vi "Configure Calculation.vi"(4 "Upper Limit Value (0)":dbl format="%#_11g", 6 "Lower Limit Value (0)":dbl format="%#_11g", 7 "Enable Statistics (Disable)":bool, 8 "error in (no error)":errorcluster, 9 "Enable Limit Filter (Disable)":bool, 10 "N (100)":i32=100 min=2 max=1000000, 11 "VISA resource name":refnum<visa-resource-name>) -> (0 "error out":errorcluster, 3 "VISA resource name out":refnum<visa-resource-name>)   [LabVIEW 2020, in "Counter.lvlib" / "PICOTEST U62XXA series.lvlib"]
doc: "Configures settings required for post-acquisition Statistics computation.\n\n<B>Note:</B>\n\nTotalize and Volt Peak Measurements <B>does not</B> support post acquisiton Statistics computation."
uses:
  PICOTEST U62XXA series.lvlib
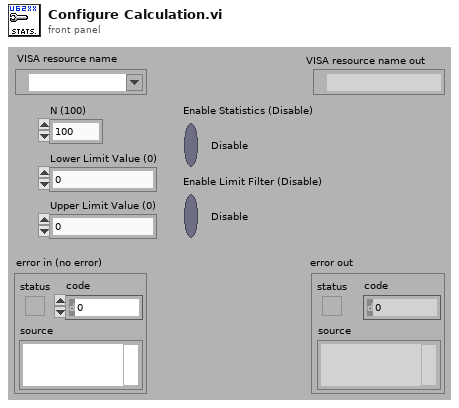
[diagram p1: front panel]
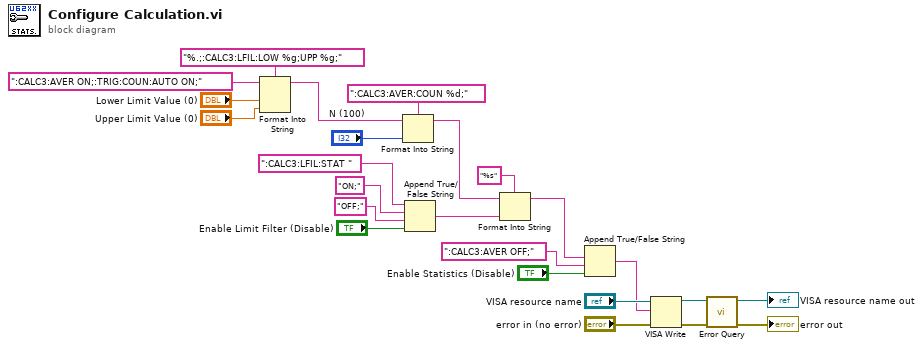
[diagram p0: block diagram]
diagram:
  n1 = Format Into String(format string="%.;:CALC3:LFIL:LOW %g;UPP %g;", initial string=":CALC3:AVER ON;:TRIG:COUN:AUTO ON;" ("format string"), "Lower Limit Value (0)", "Upper Limit Value (0)") -> (resulting string=w5:string)  [unwired: 1 in, 1 out]
  n2 = Format Into String(format string=":CALC3:AVER:COUN %d;", initial string=w5, "N (100)") -> (resulting string=w4:string)  [unwired: 1 in, 1 out]
  n3 = Append True/False String(1:"Enable Limit Filter (Disable)", 2:"OFF;" ("multi-line string"), 3:"ON;" ("multi-line string"), 4:":CALC3:LFIL:STAT " ("format string")) -> (0:w3:string)
  n4 = Format Into String(format string="%s", initial string=w4, w3) -> (resulting string=w1:string)  [unwired: 1 in, 1 out]
  n5 = Append True/False String(1:"Enable Statistics (Disable)", 2:":CALC3:AVER OFF;" ("string (\"\")"), 3:w1) -> (0:w7:string)  [unwired: 1 in]
  n6 = VISA Write(VISA resource name="VISA resource name", write buffer=w7, error in (no error)="error in (no error)") -> (VISA resource name out=w17:refnum<visa-resource-name>, error out=w16:errorcluster)  [unwired: 1 out]
  n7 = call "Error Query.vi"("error in (no error)"=w16, "VISA resource name"=w17) -> ("error out"=→"error out":errorcluster, "VISA resource name out"=→"VISA resource name out":refnum<visa-resource-name>)  [unwired: 6 in, 2 out]
